vi "Save Cursors.vi"(0 "Display State In":T1, 5 "Path":path, 9 "Container State":T2, 11 "error in (no error)":errorcluster) -> (4 "Display State Out":T1, 15 "error out":errorcluster)   [LabVIEW 2014, in "Graph with cursors XControl.xctl"]
uses:
  Graph with cursors XControl.xctl
  <vilib>/_xctls/Container State.ctl
  Graph with cursors State.ctl
  <vilib>/_xctls/XControlSupport.lvlib
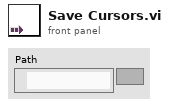
[diagram p1: front panel]
types:
  T1 = typedef "Graph with cursors XControl.xctl/Graph with cursors State.ctl" = cluster{"Cursor names":string[], "Cursor positions":dbl[], "Cursor pairs":i32, "Graph":refnum<vi>, "Prefix":string, "Base path":path}
  T2 = typedef "XControlSupport.lvlib/Container State.ctl" = cluster{"Indicator?":bool, "Run Mode?":bool, " Refnum":refnum<vi>}
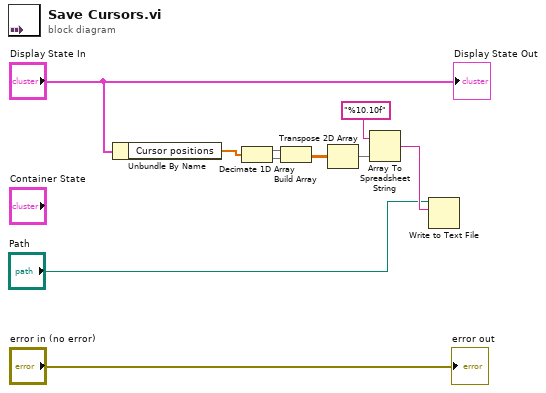
[diagram p0: block diagram]
diagram:
  n1 = Unbundle By Name("Display State In") -> ("Cursor positions"=w8:dbl[])
  n2 = Decimate 1D Array(w8) -> (w7:dbl[], w6:dbl[])
  n3 = Build Array(w7, w6) -> (w2:dbl[][])
  n4 = Transpose 2D Array(2D array=w2) -> (transposed array=w1:dbl[][])
  n5 = Array To Spreadsheet String(array=w1, 3:"%10.10f" ("format string")) -> (spreadsheet string=w4:string)  [unwired: 1 in]
  n6 = Write to Text File(file (use dialog)="Path", text=w4) -> ()  [unwired: 2 in, 3 out]
  "Display State Out" <- "Display State In"
  "error out" <- "error in (no error)"
